vi "Broadcast Centrifuge Settings.vi"(8 "error in (no error)":errorcluster, 10 "Message Queues":T6, 11 "Pump Module Config":T1={"GUID"="", "Drop Coords"={"Horizontal"=0, "Vertical"=0}, "Process Name"="", "User name"="", "Queue Name"="", "Settings"={"Cycle Period"=500.0, "Manual Entry"=0.0, "Output Device"=enum."Default", "EPOS4 Settings"={"VISA resource name"="", "axis"={"keyHandle"=1, "nodeId"=1}, "Simulated?"=TRUE}}, "Load Count"=0}) -> (0 "error out":errorcluster)   [LabVIEW 2018, in "Centrifuge Module.lvlib"]
uses:
  Centrifuge Module.lvlib
  All Message Queues.ctl
  support/Message Queue/Message Cluster.ctl
  Centrifuge Module Config Cluster.ctl
  <vilib>/Utility/miscctls.llb/LVPoint32TypeDef.ctl
  Centrifuge Module Settings Cluster.ctl
  EPOS4/Controls/Device Selection.ctl
  EPOS4/Controls/EPOS Communication Settings.ctl
  support/Message Queue/Enqueue Message (Single).vi
  support/Message Queue/Message Queue.lvlib
  EPOS4/EPOS4.lvlib
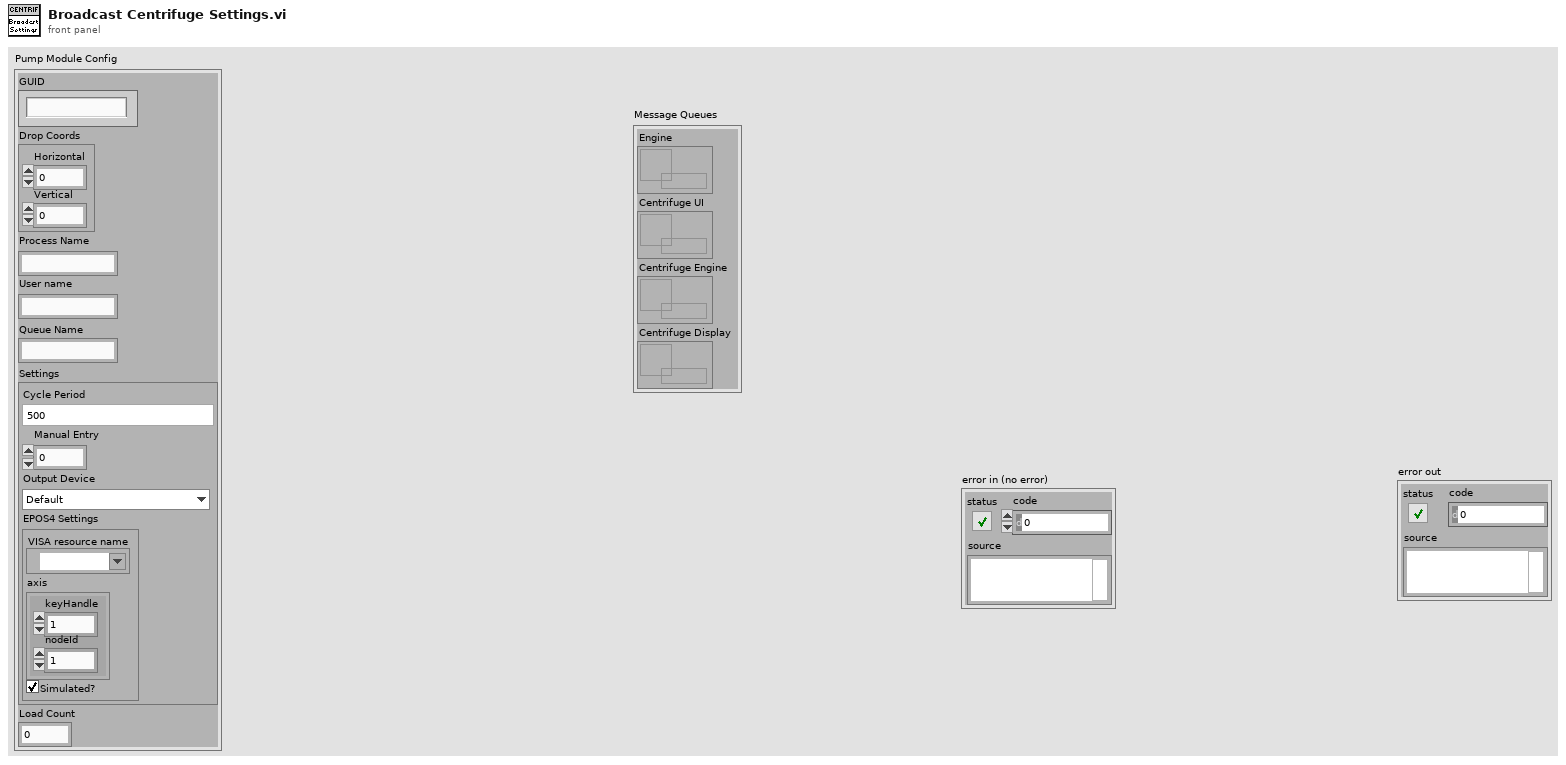
[diagram p1: front panel]
types:
  T1 = typedef "Centrifuge Module.lvlib/Centrifuge Module Config Cluster.ctl" = cluster{"GUID":string, "Drop Coords":T2, "Process Name":string, "User name":string, "Queue Name":string, "Settings":T3, "Load Count":i32}
  T2 = typedef "LVPoint32TypeDef.ctl" = cluster{"Horizontal":i32, "Vertical":i32}
  T3 = typedef "Centrifuge Module.lvlib/Centrifuge Module Settings Cluster.ctl" = cluster{"Cycle Period":dbl, "Manual Entry":dbl, "Output Device":T4, "EPOS4 Settings":T5}
  T4 = typedef "Device Selection.ctl" = enum16{"Default", "EPOS4"}
  T5 = typedef "EPOS4.lvlib/EPOS Communication Settings.ctl" = cluster{"VISA resource name":refnum<visa-resource-name>, "axis":cluster{"keyHandle":u32, "nodeId":u16}, "Simulated?":bool}
  T6 = typedef "Centrifuge Module.lvlib/All Message Queues.ctl" = cluster{"Engine":refnum<queue>, "Centrifuge UI":refnum<queue>, "Centrifuge Engine":refnum<queue>, "Centrifuge Display":refnum<queue>}
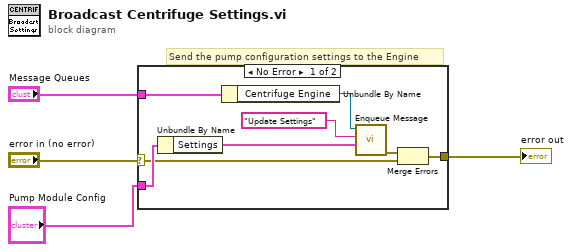
[diagram p0: block diagram]
diagram:
  # "Send the pump configuration settings to the Engine"
  n1 = case shown="No Error" "error in (no error)" {
    selector: "error in (no error)" -> [w10 w13]
    tunnel: [w12 w13] -> w2
    tunnel: "Pump Module Config" -> [w11 _]
    tunnel: "Message Queues" -> [w9 _]
    frame No Error {
      n2 = Unbundle By Name(w11) -> ("Settings"=w5:T3)
      n3 = Unbundle By Name(w9) -> ("Centrifuge Engine"=w8:refnum<queue>)
      n4 = call-poly "Enqueue Message.vi"("Message Data"=w5, "Message"="Update Settings", "Message Queue"=w8) -> ("error out"=w7:errorcluster)  [unwired: 7 in, 1 out]
      n5 = Merge Errors(w7, w10) -> (w12:errorcluster)
    }
    frame Error {
    }
  }
  "error out" <- w2
